vi "ButtonMotorControl.vi"(6 "Reverse Direction?":bool, 8 "Rev Config":T2={"Rev Power"=0.0, "Rev Press and Hold?"=TRUE} {"Rev Power" scale=0.0..1.0}, 9 "Fwd Config":T3={"Fwd Power"=0.0, "Fwd Press and Hold?"=TRUE} {"Fwd Power" scale=0.0..1.0}, 10 "Input":cluster{"Fwd Input":bool, "Rev Input":bool}, 11 "Motor Name":string) -> ()   [LabVIEW 2016]
uses:
  Control 1.ctl
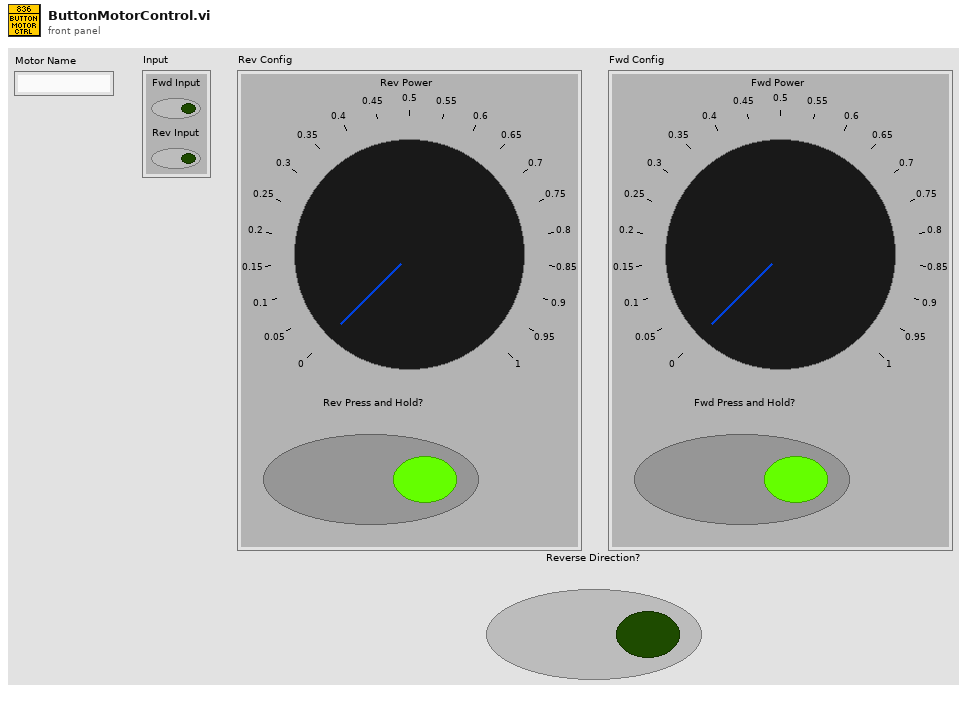
[diagram p1: front panel]
types:
  T1 = typedef "Control 1.ctl" = bool
  T2 = cluster{"Rev Power":dbl, "Rev Press and Hold?":T1}
  T3 = cluster{"Fwd Power":dbl, "Fwd Press and Hold?":T1}
  T4 = typedef "WPI_MotorControlDeviceRef.ctl" = cluster{"DeviceStatus":errorcluster, "Type":T5, "PWM":cluster{"PWM Channel":T6, "DeadBand":T7}, "CAN":cluster{"Device Number":u8, "SetOutput VI Ref":variant, "GetOutput VI Ref":variant, "Enable VI Ref":variant, "Disable VI Ref":variant, "Data":variant}, "Invert":bool}
  T5 = typedef "WPI_MotorControlType.ctl" = enum16{"PWM", "CAN"}
  T6 = typedef "FPGA_DIOPWMChannel.ctl" = enum8{"PWM 0", "PWM 1", "PWM 2", "PWM 3", "PWM 4", "PWM 5", "PWM 6", "PWM 7", "PWM 8", "PWM 9", "PWM MXP 0", "PWM MXP 1", "PWM MXP 2", "PWM MXP 3", "PWM MXP 4", "PWM MXP 5", "PWM MXP 6", "PWM MXP 7", "PWM MXP 8", "PWM MXP 9", "Invalid"}
  T7 = typedef "WPI_PWMDeadband.ctl" = cluster{"Name":string, "maxPositivePwm":i32, "minPositivePwm":i32, "centerPwm":i32, "maxNegativePwm":i32, "minNegativePwm":i32, "angularRange":u16}
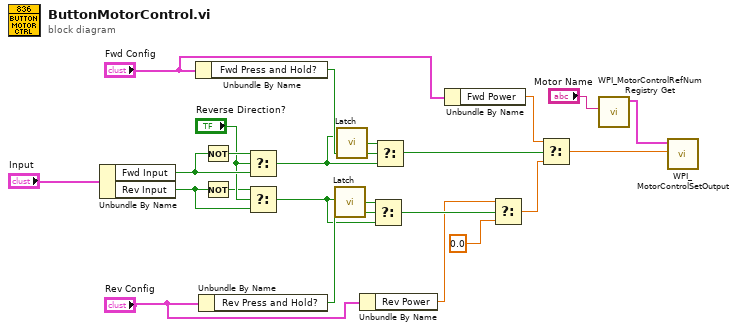
[diagram p0: block diagram]
diagram:
  n1 = Unbundle By Name("Input") -> ("Fwd Input"=w22:bool, "Rev Input"=w18:bool)
  n2 = Unbundle By Name("Fwd Config") -> ("Fwd Press and Hold?"=w17:T1)
  n3 = Unbundle By Name("Rev Config") -> ("Rev Press and Hold?"=w14:T1)
  n4 = Not(x=w22) -> (.not. x?=w21:bool)
  n5 = Not(x=w18) -> (.not. x?=w19:bool)
  n6 = Select(t=w21, s="Reverse Direction?", f=w22) -> (s? t:f=w15:bool)
  n7 = Select(t=w19, s="Reverse Direction?", f=w18) -> (s? t:f=w12:bool)
  n8 = call <userlib>:"Latch.vi"("In"=w12) -> ("Out"=w13:bool)  [unwired: 1 in]
  n9 = call <userlib>:"Latch.vi"("In"=w15) -> ("Out"=w16:bool)  [unwired: 1 in]
  n10 = Unbundle By Name("Rev Config") -> ("Rev Power"=w5:dbl)
  n11 = Select(t=w13, s=w14, f=w12) -> (s? t:f=w7:bool)
  n12 = Select(t=w16, s=w17, f=w15) -> (s? t:f=w10:bool)
  n13 = Unbundle By Name("Fwd Config") -> ("Fwd Power"=w9:dbl)
  n14 = Select(t=w5, s=w7, f=0.0) -> (s? t:f=w8:dbl)
  n15 = Select(t=w9, s=w10, f=w8) -> (s? t:f=w3:dbl)
  n16 = call <vilib>:"WPI_MotorControlRefNum Registry Get.vi"("refnum name"="Motor Name") -> ("MotorControlDevRef"=w2:T4)  [unwired: 9 in, 1 out]
  n17 = call <vilib>:"WPI_MotorControlSetOutput.vi"("Output"=w3, "MotorControlDevRef"=w2) -> ()  [unwired: 7 in, 3 out]
